vi "Read.vi"(8 "error in (no error)":errorcluster, 11 "Serial in":refnum<class "Serial.lvclass">) -> (0 "error out":errorcluster, 2 "Read":string, 3 "Serial out":refnum<class "Serial.lvclass">)   [LabVIEW 2021, in "Communication.lvlib" / "Serial.lvclass"]
uses:
  Serial.lvclass
  Serial.lvclass/Serial.ctl
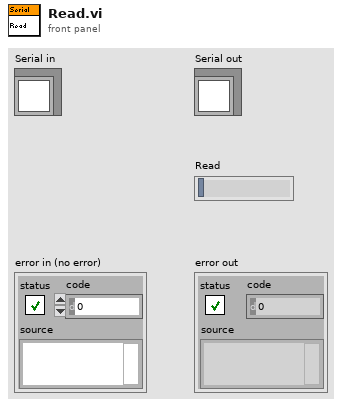
[diagram p1: front panel]
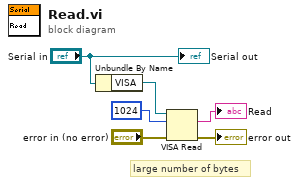
[diagram p0: block diagram]
diagram:
  # "large number of bytes"
  n1 = Unbundle By Name("Serial in") -> ("VISA"=w2:refnum<visa-resource-name>)
  n2 = VISA Read(VISA resource name=w2, byte count=u32 1024, error in (no error)="error in (no error)") -> (read buffer=→"Read":string, error out=→"error out":errorcluster)  [unwired: 2 out]
  "Serial out" <- "Serial in"
